vi "vipm_BuildDailyVIP.vi"(8 "error in (no error)":errorcluster, 11 "CommandLine":string[](array[string])) -> (0 "error out":errorcluster, 2 "test details":string, 3 "output to action":string)   [LabVIEW 2014]
uses:
  <userlib>/_OpenG.lib/file/file.llb/File Exists - Scalar__ogtk.vi
  <userlib>/_OpenG.lib/string/string.llb/Trim Whitespace (String)__ogtk.vi
  <vilib>/JKI/VIPM API/VIPM API_vipm_api.lvlib
  _lvcicd/_lvcicd_support_2014.lvlib
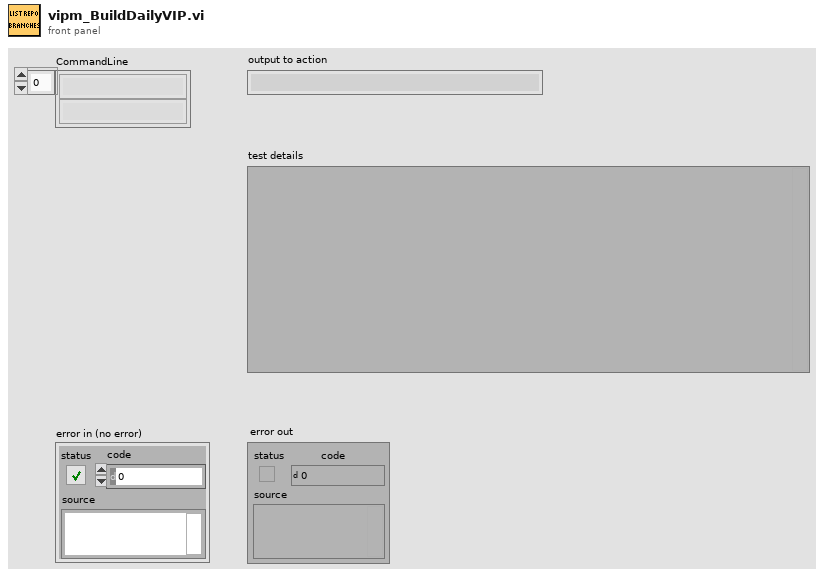
[diagram p1: front panel]
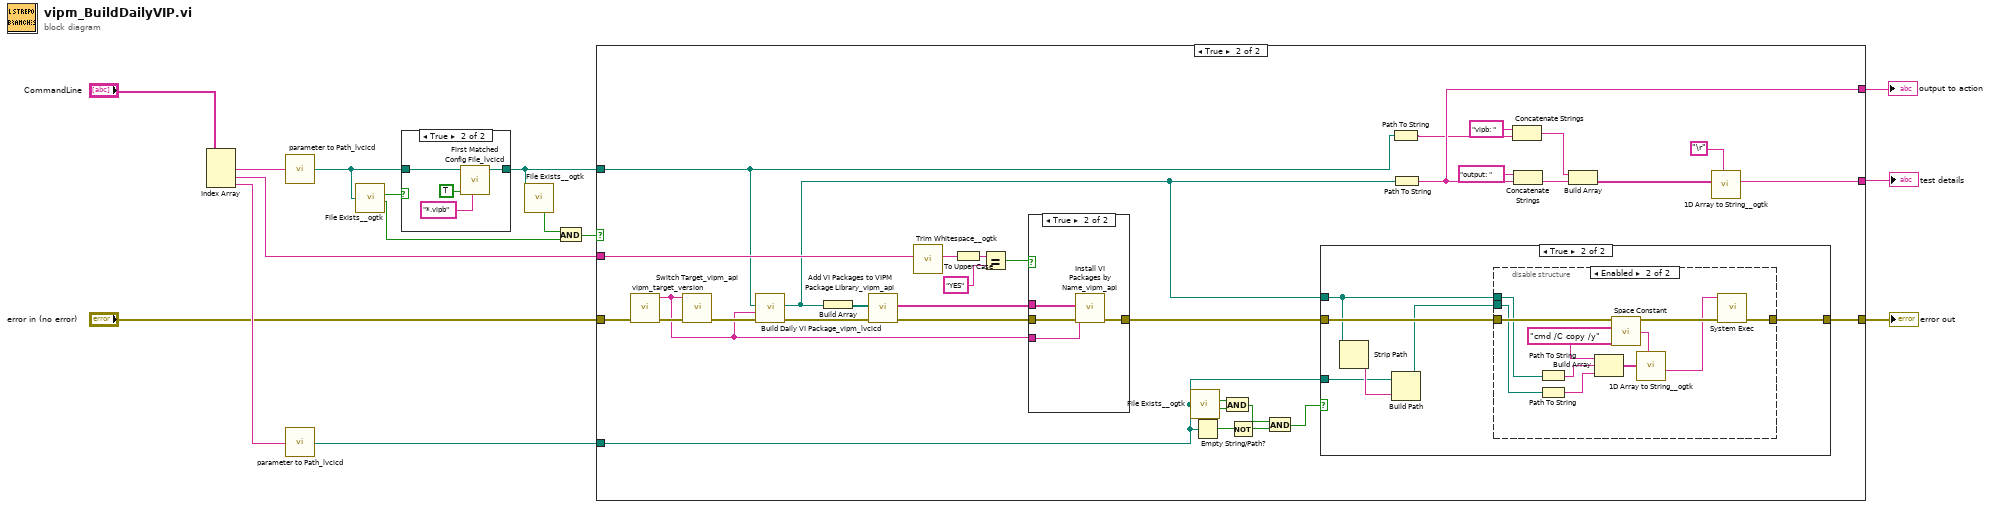
[diagram p0: block diagram]
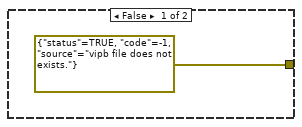
[diagram p3: hidden frame]
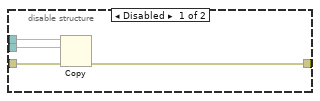
[diagram p5: hidden frame]
diagram:
  n1 = Index Array(array="CommandLine") -> (element #1=w14:string, element #2=w13:string, element #3=w11:string)  [unwired: 3 in]
  n2 = call "parameter to Path_lvcicd.vi"("String"=w14) -> ("Path"=w7:path)
  n3 = call "parameter to Path_lvcicd.vi"("String"=w11) -> ("Path"=w12:path)
  n4 = call-poly <userlib>:"File Exists__ogtk.vi"("file path"=w7) -> ("is directory"=w6:bool, "exists"=w4:bool)  [unwired: 6 in]
  n5 = case shown="True" w6 {
    tunnel: w7 -> [w16 w19]
    tunnel: [w16 w18] -> w2
    frame False {
    }
    frame True {
      n6 = call "First Matched Config File_lvcicd.vi"("pattern(ini by default)"="*.vipb", "Recrusively(F)"=TRUE, "Searching Directory"=w19) -> ("Matched Config File"=w18:path)  [unwired: 8 in]
    }
  }
  n7 = call-poly <userlib>:"File Exists__ogtk.vi"("file path"=w2) -> ("exists"=w5:bool)  [unwired: 6 in, 1 out]
  n8 = And(x=w5, y=w4) -> (x .and. y?=w3:bool)
  n9 = case shown="True" w3 {
    tunnel: w13 -> [_ w47]
    tunnel: w12 -> [_ w43]
    tunnel: [errorcluster {"status"=TRUE, "code"=-1, "source"="vipb file does not exists."} ("error out") w42] -> w10
    tunnel: "error in (no error)" -> [_ w34]
    tunnel: [_ w23] -> w8
    tunnel: w2 -> [_ w26]
    tunnel: [_ w31] -> w1
    frame False {
    }
    frame True {
      n10 = call "vipm_target_version.vi"() -> ("vipm Taget version"=w32:string)  [unwired: 11 in]
      n11 = call <vilib>:"Switch Target_vipm_api.vi"("error in (no error)"=w34, "LabVIEW Version"=w32) -> ("error out"=w33:errorcluster)  [unwired: 9 in]
      n12 = call "Build Daily VI Package_vipm_lvcicd.vi"("error in (no error)"=w33, "LabVIEW Version"=w32, "vipb"=w26) -> ("error out"=w52:errorcluster, "Build Output"=w41:path)  [unwired: 5 in, 2 out]
      n13 = Build Array(w41) -> (w53:path[])
      n14 = call <vilib>:"Add VI Packages to VIPM Package Library_vipm_api.vi"("error in (no error)"=w52, "Packages to add to VIPM Library (vipc,vip,ogp)"=w53) -> ("error out"=w51:errorcluster, "Package Names Added"=w50:string[])  [unwired: 8 in]
      n15 = call-poly <userlib>:"Trim Whitespace__ogtk.vi"("String in"=w47) -> ("String out"=w44:string)  [unwired: 6 in]
      n16 = To Upper Case(1:w44) -> (0:w45:string)
      n17 = Equal?(x=w45, y="YES") -> (x = y?=w48:bool)
      n18 = case shown="True" w48 {
        tunnel: w51 -> [w75 w79]
        tunnel: [w75 w78] -> w49
        tunnel: w32 -> [_ w77]
        tunnel: w50 -> [_ w76]
        frame False {
        }
        frame True {
          n19 = call <vilib>:"Install VI Packages by Name_vipm_api.vi"("error in (no error)"=w79, "LabVIEW Version"=w77, "Package Names to Install []"=w76) -> ("error out"=w78:errorcluster)  [unwired: 8 in]
        }
      }
      n20 = call-poly <userlib>:"File Exists__ogtk.vi"("file path"=w43) -> ("is directory"=w40:bool, "exists"=w39:bool)  [unwired: 6 in]
      n21 = Empty String/Path?(string/path=w43) -> (empty?=w38:bool)
      n22 = And(x=w40, y=w39) -> (x .and. y?=w37:bool)
      n23 = Not(x=w38) -> (.not. x?=w35:bool)
      n24 = And(x=w37, y=w35) -> (x .and. y?=w36:bool)
      n25 = case shown="True" w36 {
        tunnel: w49 -> [w54 w60]
        tunnel: [w54 w59] -> w42
        tunnel: w41 -> [_ w57]
        tunnel: w43 -> [_ w55]
        frame False {
        }
        frame True {
          n26 = Strip Path(path=w57) -> (name=w56:string)  [unwired: 1 out]
          n27 = Build Path(base path=w55, name or relative path=w56) -> (appended path=w58:path)
          n28 = disable-structure shown="Enabled" {
            disable-tunnel: w60 -> [w64 w73]
            disable-tunnel: [w63 w74] -> w59
            disable-tunnel: w58 -> [w62 w71]
            disable-tunnel: w57 -> [w61 w72]
            frame Disabled {
              n29 = Copy(8:w64, 10:w62, 11:w61) -> (0:w63:errorcluster)  [unwired: 2 in, 2 out]
            }
            frame Enabled {
              n30 = Path To String(path=w72) -> (string=w69:string)
              n31 = Path To String(path=w71) -> (string=w68:string)
              n32 = Build Array("cmd /C copy /y" ("name"), w69, w68) -> (w67:string[])
              n33 = call <vilib>:"Space Constant.vi"() -> ("String"=w66:string)
              n34 = call <userlib>:"1D Array to String__ogtk.vi"("delimiter (Tab)"=w66, "Array of Strings"=w67) -> ("delimited string"=w65:string)  [unwired: 9 in]
              n35 = call <vilib>:"System Exec.vi"("error in (no error)"=w73, "command line"=w65) -> ("error out"=w74:errorcluster)  [unwired: 6 in, 3 out]
            }
          }
        }
      }
      n36 = Path To String(path=w26) -> (string=w27:string)
      n37 = Path To String(path=w41) -> (string=w31:string)
      n38 = Concatenate Strings("vipb: " ("string"), w27) -> (w24:string)
      n39 = Concatenate Strings("output: " ("string"), w31) -> (w30:string)
      n40 = Build Array(w24, w30) -> (w25:string[])
      n41 = call <userlib>:"1D Array to String__ogtk.vi"("delimiter (Tab)"="\r", "Array of Strings"=w25) -> ("delimited string"=w23:string)  [unwired: 9 in]
    }
  }
  "test details" <- w8
  "error out" <- w10
  "output to action" <- w1
